vi "TDC数据处理_32b.vi"(6 "存储文件路径":path=path "C:/Users/Lebron/Desktop/tdc测试数据/Plain3/10ns.txt", 7 "路径":path caption="文件路径 （空时为对话框）") -> (0 "时间分布谱":dbl[](graph), 1 "b细计数分布谱":dbl[](graph), 2 "a细计数分布谱":dbl[](graph))   [LabVIEW 2014]
uses:
  <vilib>/Utility/file.llb/Read From Spreadsheet File (DBL).vi
  <vilib>/Utility/file.llb/Write To Spreadsheet File (DBL).vi
panel:
  out "ax细计数":i32[](array[numeric])
  out "粗计数":i32[](array[numeric])
  out "粗计数2分布":dbl[](graph)
  out "粗计数1分布":dbl[](graph)
  out "粗计数1分布谱":dbl[](graph)
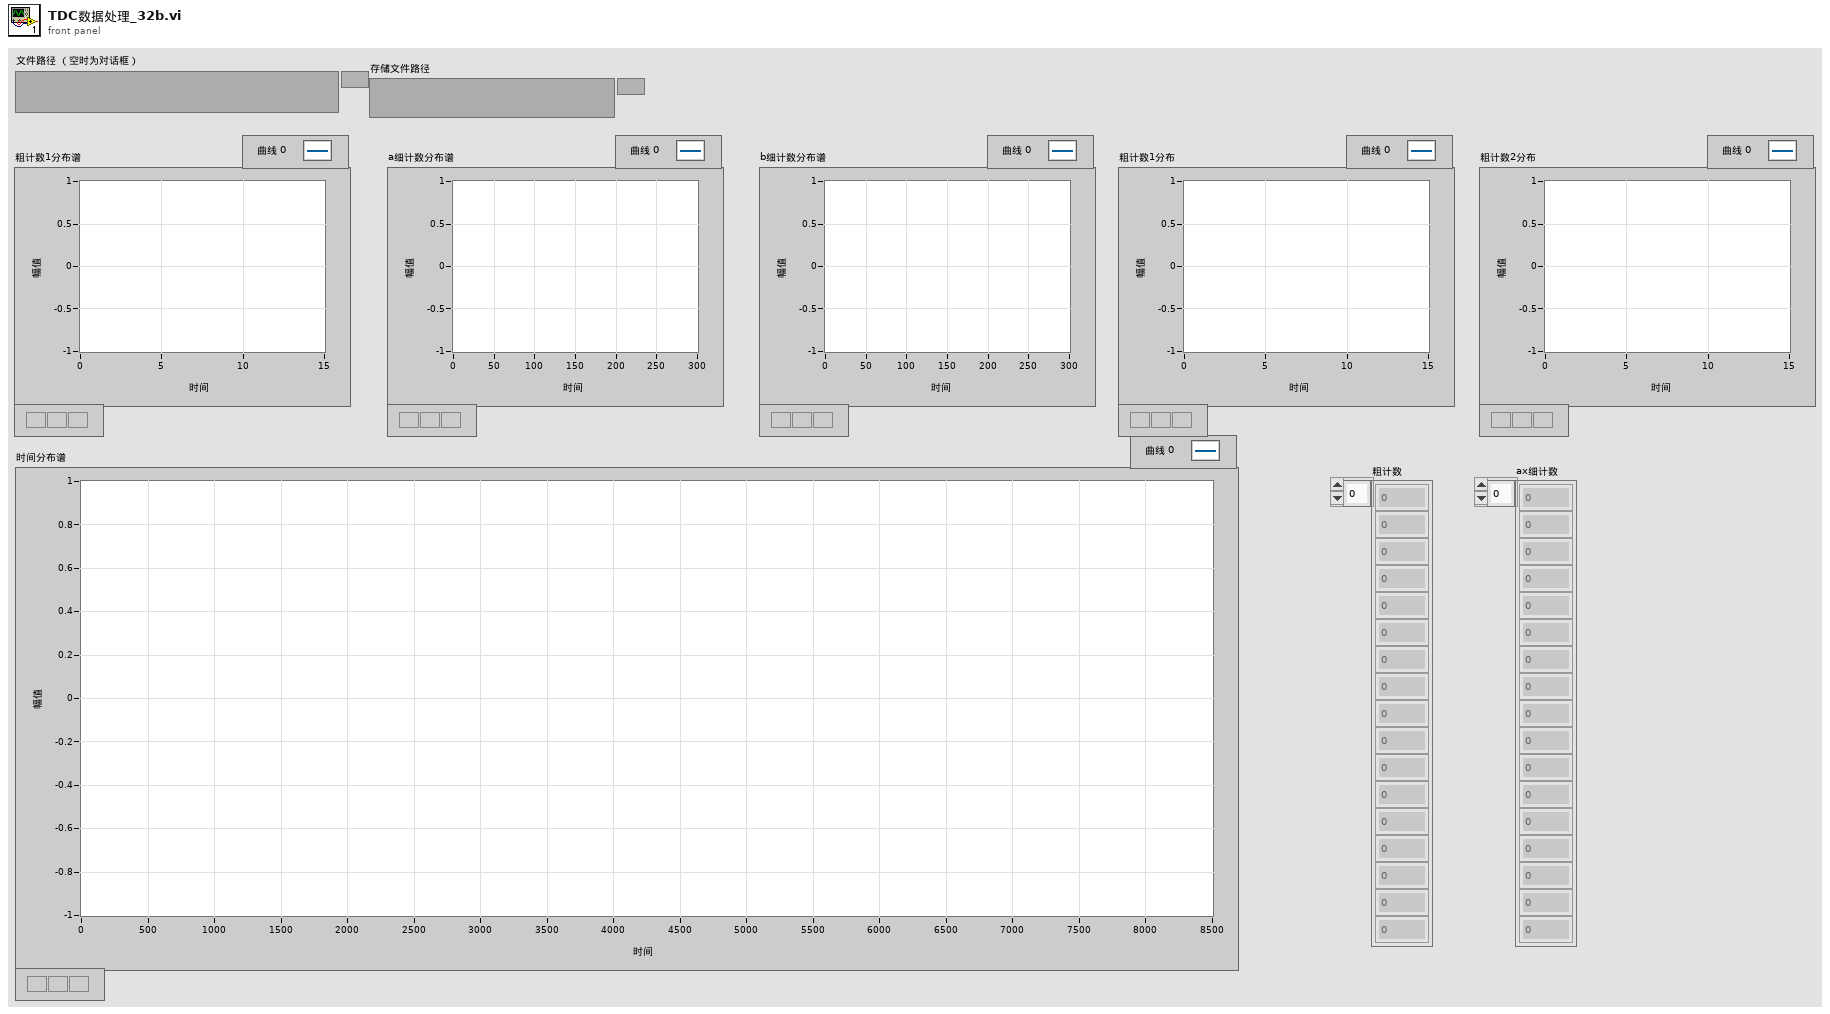
[diagram p1: front panel]
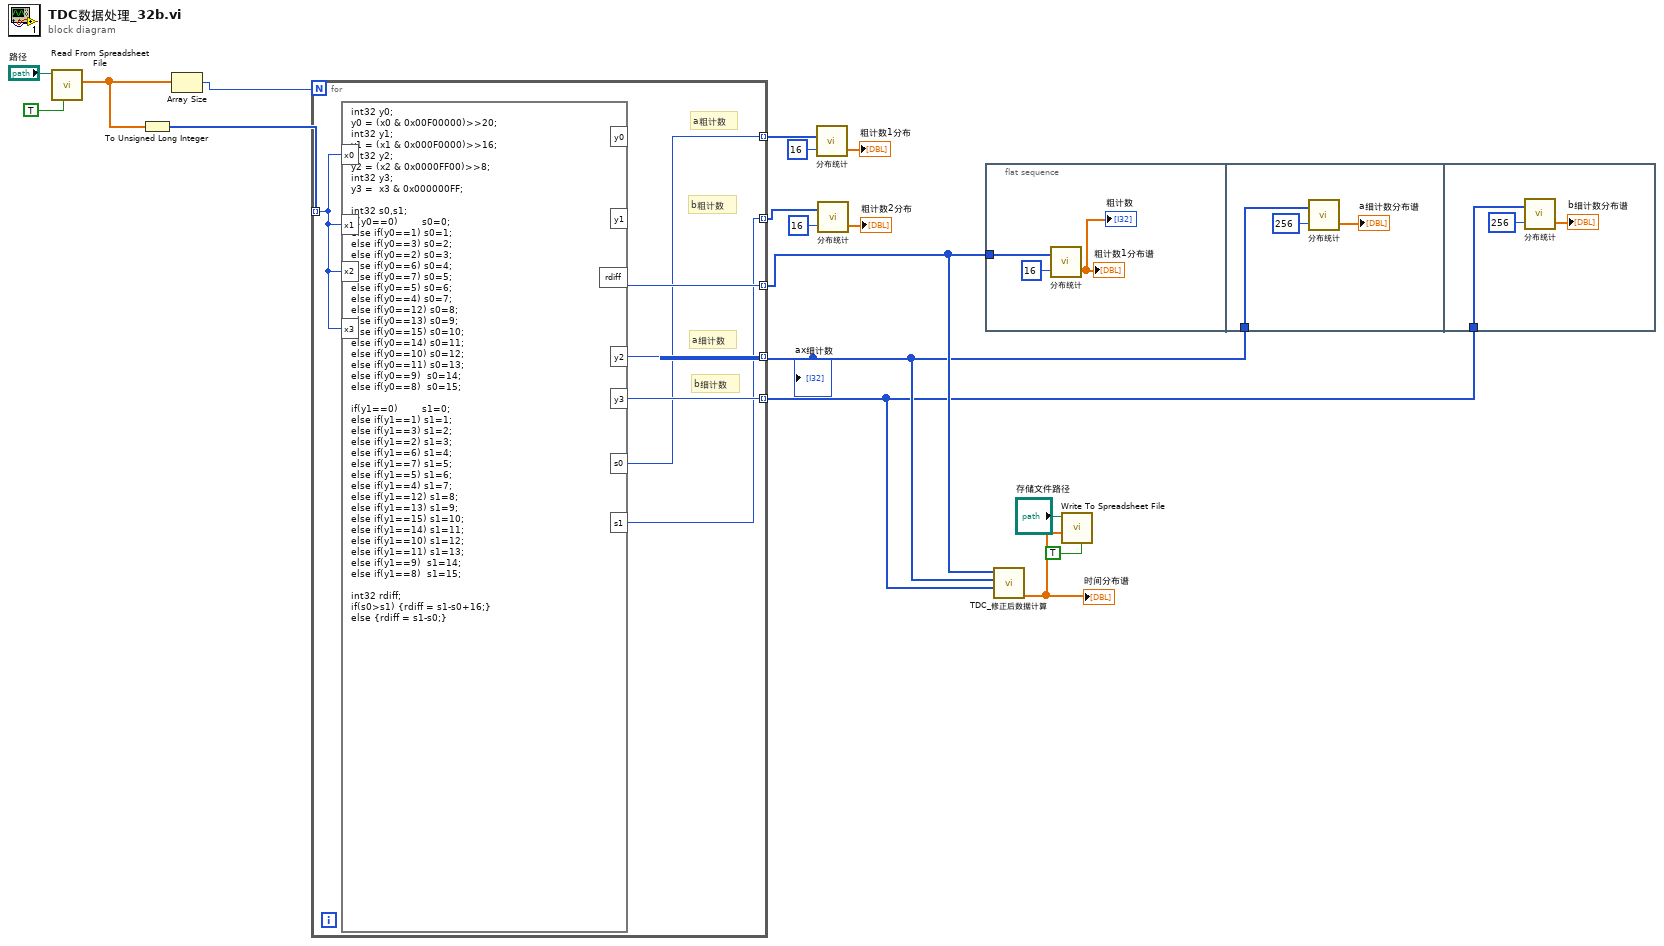
[diagram p0: block diagram]
diagram:
  n1 = call-poly <vilib>:"Read From Spreadsheet File.vi"("transpose (no:F)"=TRUE, "file path (dialog if empty)"="路径") -> ("first row"=w15:dbl[])  [unwired: 5 in, 4 out]
  n2 = To Unsigned Long Integer(number=w15) -> (unsigned 32bit integer=w13:u32[])
  n3 = Array Size(array=w15) -> (size(s)=w14:i32)
  n4 = for {
    N: w14 -> [_]
    tunnel: w13 -> [w21] mode=indexing
    tunnel: [w18] -> w6 mode=indexing
    tunnel: [w23] -> w11 mode=indexing
    tunnel: [w22] -> w10 mode=indexing
    tunnel: [w19] -> w9 mode=indexing
    tunnel: [w20] -> w12 mode=indexing
    # "a粗计数"
    # "a细计数"
    # "b细计数"
    # "b粗计数"
    n5 = formula code="int32 y0;\ny0 = (x0 & 0x00F00000)>>20;\nint32 y1;\ny1 = (x1 & 0x000F0000)>>16;\nint32 y2;\ny2 = (x2 & 0x0000FF00)>>8;\nint32 y3;\ny3 =  x3 & 0x000000FF;\n\nint32 s0,s1;\nif(y0==0)        s0=0;\nelse if(y0==1) s0=1;\nelse if(y0==3) s0=2;\nelse if(y0==2) s0=3;\nelse if(y0==6) s0=4;\nelse if(y0==7) s0=5;\nelse if(y0==5) s0=6;\nelse if(y0==4) s0=7;\nelse if(y0==12) s0=8;\nelse if(y0==13) s0=9;\nelse if(y0==15) s0=10;\nelse if(y0==14) s0=11;\nelse if(y0==10) s0=12;\nelse if(y0==11) s0=13;\nelse if(y0==9)  s0=14;\nelse if(y0==8)  s0=15;\n\nif(y1==0)        s1=0;\nelse if(y1==1) s1=1;\nelse if(y1==3) s1=2;\nelse if(y1==2) s1=3;\nelse if(y1==6) s1=4;\nelse if(y1==7) s1=5;\nelse if(y1==5) s1=6;\nelse if(y1==4) s1=7;\nelse if(y1==12) s1=8;\nelse if(y1==13) s1=9;\nelse if(y1==15) s1=10;\nelse if(y1==14) s1=11;\nelse if(y1==10) s1=12;\nelse if(y1==11) s1=13;\nelse if(y1==9)  s1=14;\nelse if(y1==8)  s1=15;\n\nint32 rdiff;\nif(s0>s1) {rdiff = s1-s0+16;}\nelse {rdiff = s1-s0;}"("x1"=w21, "x2"=w21, "x3"=w21, "x0"=w21) -> ("y2"=w23:i32, "y3"=w22:i32, "rdiff"=w20:i32, "s0"=w19:i32, "s1"=w18:i32)  [unwired: 2 out]
  }
  "ax细计数" <- w11
  n6 = call "分布统计.vi"("道数"=16, "数组"=w9) -> ("分布谱"=→"粗计数1分布":dbl[])  [unwired: 1 out]
  n7 = call "分布统计.vi"("道数"=16, "数组"=w6) -> ("分布谱"=→"粗计数2分布":dbl[])  [unwired: 1 out]
  n8 = flat-sequence {
    tunnel: w12 -> [w25]
    tunnel: w11 -> [w29]
    tunnel: w10 -> [w32]
    frame #0 {
      n9 = call "分布统计.vi"("道数"=16, "数组"=w25) -> ("分布谱"=→"粗计数1分布谱" →"粗计数":dbl[])  [unwired: 1 out]
    }
    frame #1 {
      n10 = call "分布统计.vi"("道数"=256, "数组"=w29) -> ("分布谱"=→"a细计数分布谱":dbl[])  [unwired: 1 out]
    }
    frame #2 {
      n11 = call "分布统计.vi"("道数"=256, "数组"=w32) -> ("分布谱"=→"b细计数分布谱":dbl[])  [unwired: 1 out]
    }
  }
  n12 = call "TDC_修正后数据计算.vi"("细计数输入2"=w10, "细计数输入1"=w11, "粗计数"=w12) -> ("分布谱"=w3:dbl[])
  "时间分布谱" <- w3
  n13 = call-poly <vilib>:"Write To Spreadsheet File.vi"("transpose? (no:F)"=TRUE, "1D data"=w3, "file path (dialog if empty)"="存储文件路径") -> ()  [unwired: 5 in, 1 out]
